vi "UIntToLittleEndian.vi"(9 "Number":u32=1000) -> (1 "byte array":u8[](array[numeric])=[0, 0, 232, 3] format="%x")   [LabVIEW 2009]
panel:
  out "string":string
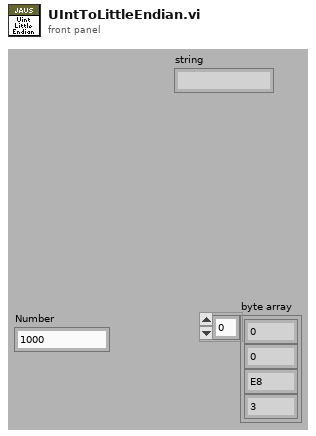
[diagram p1: front panel]
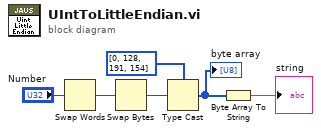
[diagram p0: block diagram]
diagram:
  n1 = Swap Words(1:"Number") -> (0:w1:u32)
  n2 = Swap Bytes(anything=w1) -> (byte swapped=w5:u32)
  n3 = Type Cast(type=u8[] [0, 128, 191, 154] ("byte array"), x=w5) -> (*(type *) &x=w3:u8[])
  "byte array" <- w3
  n4 = Byte Array To String(unsigned byte array=w3) -> (string=→"string":string)
